vi "查询开关信息.vi"(9 "NEWS":string, 11 "TCP Network Connection in":refnum<k5>) -> (0 "error out":errorcluster, 3 "TCP Network Connection out":refnum<k5>)   [LabVIEW 2015]
uses:
  Global/SeverGlobal.vi
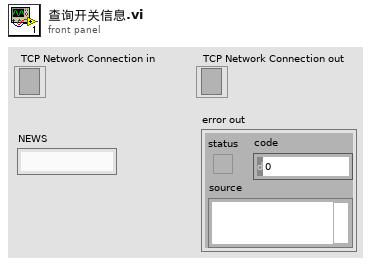
[diagram p1: front panel]
types:
  T1 = enum16{"Standard", "Buffered", "CRLF", "Immediate"}
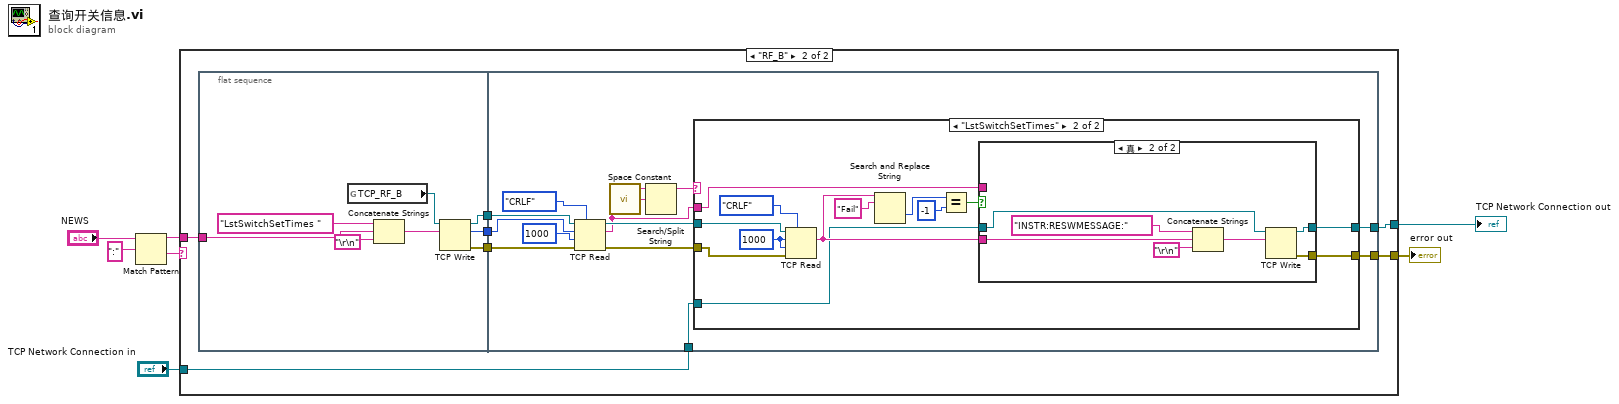
[diagram p0: block diagram]
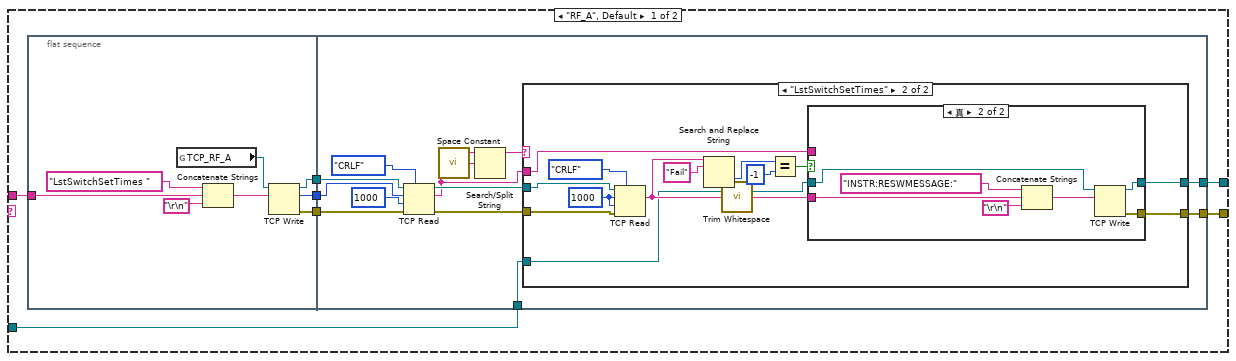
[diagram p2: hidden frame]
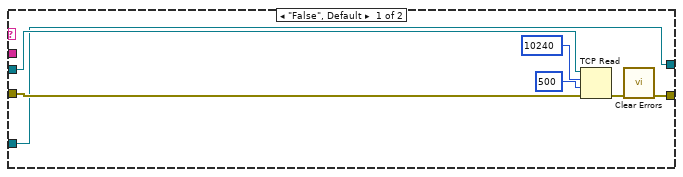
[diagram p3: hidden frame]
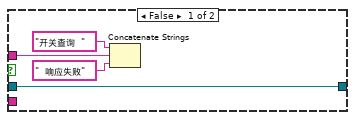
[diagram p4: hidden frame]
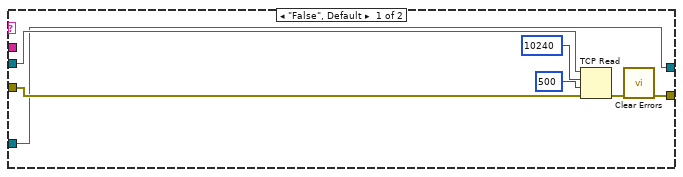
[diagram p5: hidden frame]
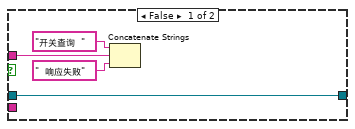
[diagram p6: hidden frame]
diagram:
  n1 = Match Pattern(string="NEWS", regular expression=":") -> (before substring=w5:string, after substring=w4:string)  [unwired: 1 in, 2 out]
  n2 = case shown="\"RF_B\"" w4 {
    tunnel: w5 -> [w14 w74]
    tunnel: "TCP Network Connection in" -> [w10 w70]
    tunnel: [w9 w69] -> w2
    tunnel: [w8 w68] -> w1
    frame "RF_A", Default {
      n3 = flat-sequence {
        tunnel: w14 -> [w20]
        tunnel: [w18] -> w13
        tunnel: [w17] -> w12
        tunnel: [w15] -> w11
        tunnel: w13 -> [w35]
        tunnel: w12 -> [w34]
        tunnel: w11 -> [w31]
        tunnel: w10 -> [w25]
        tunnel: [w24] -> w9
        tunnel: [w23] -> w8
        frame #0 {
          n4 = global read "SeverGlobal.vi" "TCP_RF_A"() -> (w22:refnum<k5>)
          n5 = Concatenate Strings("LstSwitchSetTimes " ("元素"), w20, "\r\n") -> (w19:string)
          n6 = TCP Write(connection ID=w22, data in=w19) -> (connection ID out=w18:refnum<k5>, bytes written=w15:i32, error out=w17:errorcluster)  [unwired: 2 in]
        }
        frame #1 {
          n7 = TCP Read(connection ID=w35, bytes to read=w31, error in (no error)=w34, 7:T1."CRLF" ("mode (standard)"), 9:1000 ("bytes to read")) -> (connection ID out=w28:refnum<k5>, data out=w26:string, error out=w27:errorcluster)
          n8 = call <vilib>:"Space Constant.vi"() -> ("String"=w30:string)
          n9 = Search/Split String(string=w26, search string/char (-)=w30) -> (substring before match=w29:string)  [unwired: 1 in, 2 out]
          n10 = case shown="\"LstSwitchSetTimes\"" w29 {
            tunnel: w28 -> [w40 w54]
            tunnel: w27 -> [w39 w53]
            tunnel: w26 -> [_ w48]
            tunnel: w25 -> [w37 w46]
            tunnel: [w37 w45] -> w24
            tunnel: [w36 w44] -> w23
            frame "False", Default {
              n11 = TCP Read(connection ID=w40, bytes to read=10240, error in (no error)=w39, 9:500 ("timeout ms (25000)")) -> (error out=w41:errorcluster)  [unwired: 1 in, 2 out]
              n12 = call <vilib>:"Clear Errors.vi"("error in (no error)"=w41) -> ("error out"=w36:errorcluster)  [unwired: 5 in, 1 out]
            }
            frame "LstSwitchSetTimes" {
              w56 = 1000 ("timeout ms (25000)")
              n13 = TCP Read(connection ID=w54, bytes to read=w56, error in (no error)=w53, 7:T1."CRLF" ("mode (standard)"), 9:w56) -> (data out=w47:string)  [unwired: 2 out]
              n14 = Search and Replace String(input string=w47, search string="Fail") -> (offset past replacement=w50:i32)  [unwired: 6 in, 3 out]
              n15 = call <vilib>:"Trim Whitespace.vi"("string"=w47) -> ("trimmed string"=w43:string)  [unwired: 1 in]
              n16 = Equal?(x=w50, y=-1) -> (x = y?=w49:bool)
              n17 = case shown="真" w49 {
                tunnel: w48 -> [w58 _]
                tunnel: w43 -> [_ w65]
                tunnel: w46 -> [w57 w64]
                tunnel: [w57 w62] -> w45
                tunnel: [_ w61] -> w44
                frame False {
                  n18 = Concatenate Strings("开关查询  " ("message"), w58, "  响应失败" ("message")) -> ()  [unwired: 1 out]
                }
                frame True {
                  n19 = Concatenate Strings("INSTR:RESWMESSAGE:", w65, "\r\n") -> (w63:string)
                  n20 = TCP Write(connection ID=w64, data in=w63) -> (connection ID out=w62:refnum<k5>, error out=w61:errorcluster)  [unwired: 2 in, 1 out]
                }
              }
            }
          }
        }
      }
    }
    frame "RF_B" {
      n21 = flat-sequence {
        tunnel: w74 -> [w80]
        tunnel: [w78] -> w73
        tunnel: [w77] -> w72
        tunnel: [w75] -> w71
        tunnel: w73 -> [w95]
        tunnel: w72 -> [w94]
        tunnel: w71 -> [w91]
        tunnel: w70 -> [w85]
        tunnel: [w84] -> w69
        tunnel: [w83] -> w68
        frame #0 {
          n22 = global read "SeverGlobal.vi" "TCP_RF_B"() -> (w82:refnum<k5>)
          n23 = Concatenate Strings("LstSwitchSetTimes " ("元素"), w80, "\r\n") -> (w79:string)
          n24 = TCP Write(connection ID=w82, data in=w79) -> (connection ID out=w78:refnum<k5>, bytes written=w75:i32, error out=w77:errorcluster)  [unwired: 2 in]
        }
        frame #1 {
          n25 = TCP Read(connection ID=w95, bytes to read=w91, error in (no error)=w94, 7:T1."CRLF" ("mode (standard)"), 9:1000 ("bytes to read")) -> (connection ID out=w88:refnum<k5>, data out=w86:string, error out=w87:errorcluster)
          n26 = call <vilib>:"Space Constant.vi"() -> ("String"=w90:string)
          n27 = Search/Split String(string=w86, search string/char (-)=w90) -> (substring before match=w89:string)  [unwired: 1 in, 2 out]
          n28 = case shown="\"LstSwitchSetTimes\"" w89 {
            tunnel: w88 -> [w100 w113]
            tunnel: w87 -> [w99 w112]
            tunnel: w86 -> [_ w107]
            tunnel: w85 -> [w97 w105]
            tunnel: [w97 w104] -> w84
            tunnel: [w96 w103] -> w83
            frame "False", Default {
              n29 = TCP Read(connection ID=w100, bytes to read=10240, error in (no error)=w99, 9:500 ("timeout ms (25000)")) -> (error out=w101:errorcluster)  [unwired: 1 in, 2 out]
              n30 = call <vilib>:"Clear Errors.vi"("error in (no error)"=w101) -> ("error out"=w96:errorcluster)  [unwired: 5 in, 1 out]
            }
            frame "LstSwitchSetTimes" {
              w115 = 1000 ("timeout ms (25000)")
              n31 = TCP Read(connection ID=w113, bytes to read=w115, error in (no error)=w112, 7:T1."CRLF" ("mode (standard)"), 9:w115) -> (data out=w106:string)  [unwired: 2 out]
              n32 = Search and Replace String(input string=w106, search string="Fail") -> (offset past replacement=w109:i32)  [unwired: 6 in, 3 out]
              n33 = Equal?(x=w109, y=-1) -> (x = y?=w108:bool)
              n34 = case shown="真" w108 {
                tunnel: w107 -> [w117 _]
                tunnel: w106 -> [_ w124]
                tunnel: w105 -> [w116 w123]
                tunnel: [w116 w121] -> w104
                tunnel: [_ w120] -> w103
                frame False {
                  n35 = Concatenate Strings("开关查询  " ("message"), w117, "  响应失败" ("message")) -> ()  [unwired: 1 out]
                }
                frame True {
                  n36 = Concatenate Strings("INSTR:RESWMESSAGE:", w124, "\r\n") -> (w122:string)
                  n37 = TCP Write(connection ID=w123, data in=w122) -> (connection ID out=w121:refnum<k5>, error out=w120:errorcluster)  [unwired: 2 in, 1 out]
                }
              }
            }
          }
        }
      }
    }
  }
  "error out" <- w1
  "TCP Network Connection out" <- w2
